vi "Get SMO HELP.vi"(8 "error in (no error)":errorcluster, 10 "Command":string, 11 "Instrument in":refnum<class "Instrument.lvclass">) -> (0 "error out":errorcluster, 2 "help cluster":T1, 3 "Instrument out":refnum<class "Instrument.lvclass">)   [LabVIEW 2019, in "Instrument.lvlib" / "Instrument.lvclass"]
uses:
  Instrument.lvclass
  subsystems/Help/typedefs/Help--cluster.ctl
  Typedefs/Instrument.Commands--Enum.ctl
  Typedefs/Instrument.IDN--cluster.ctl
  Typedefs/Instrument.GET--cluster.ctl
  Typedefs/Instrument.SET--cluster.ctl
  Typedefs/Instrument.HELP--Cluster.ctl
  subsystems/Help/Help.lvclass
  <vilib>/PRIrvin/JSON-Schema/JSON-Schema.lvlib
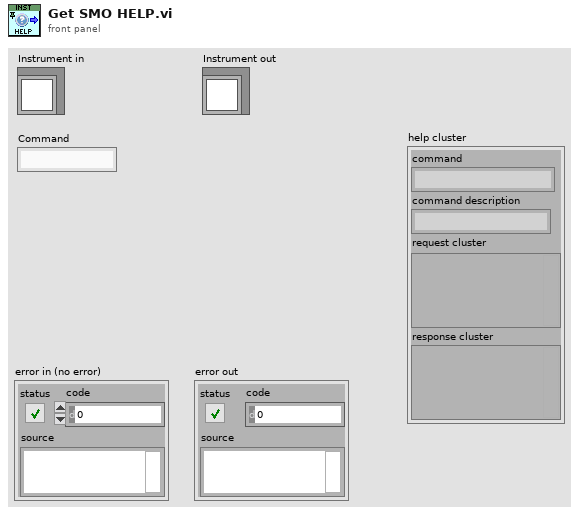
[diagram p1: front panel]
types:
  T1 = typedef "Instrument.lvlib/Help.lvclass/Help--cluster.ctl" = cluster{"command":string, "command description":string, "request cluster":variant, "response cluster":variant}
  T2 = typedef "Instrument.lvlib/Instrument.lvclass/Instrument.GET--cluster.ctl" = cluster{"parameter":string, "Data":variant}
  T3 = typedef "Instrument.lvlib/Instrument.lvclass/Instrument.SET--cluster.ctl" = cluster{"parameter":string, "Data":variant}
  T4 = typedef "Instrument.lvlib/Instrument.lvclass/Instrument.HELP--Cluster.ctl" = cluster{"command":string}
  T5 = typedef "Instrument.lvlib/Instrument.lvclass/Instrument.Commands--Enum.ctl" = enum16{"ACK", "HELP", "IDN", "getAll", "getAllData"}
  T6 = typedef "Instrument.lvlib/Instrument.lvclass/Instrument.IDN--cluster.ctl" = cluster{"vendor":string, "model":string, "serial":string, "firmware":string}
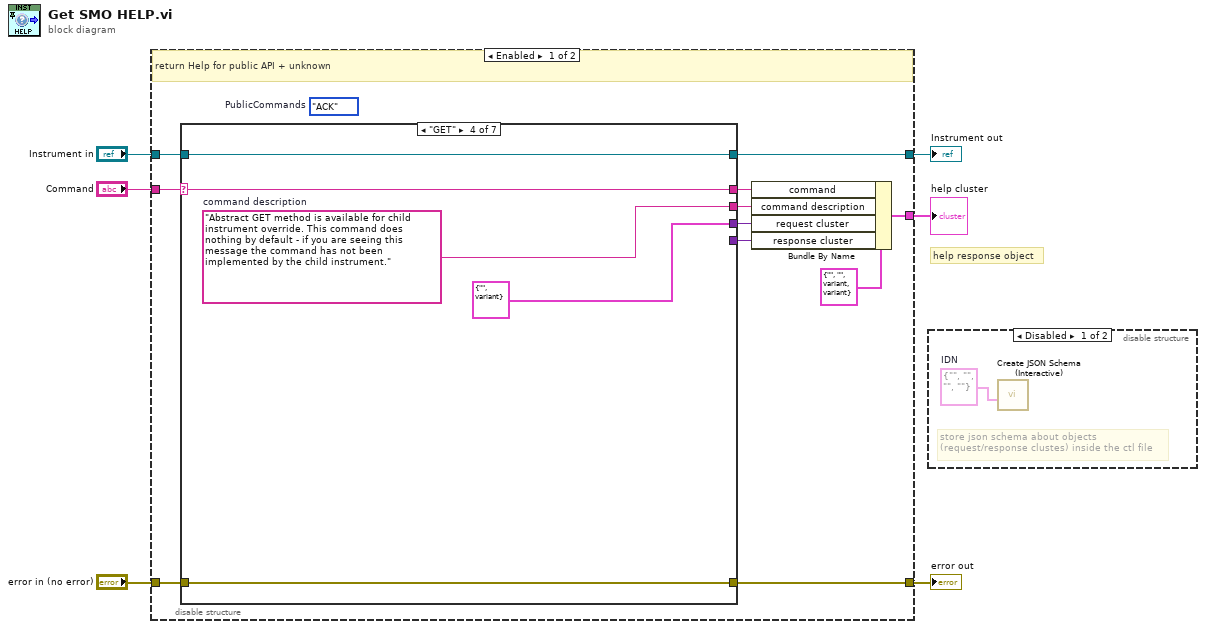
[diagram p0: block diagram]
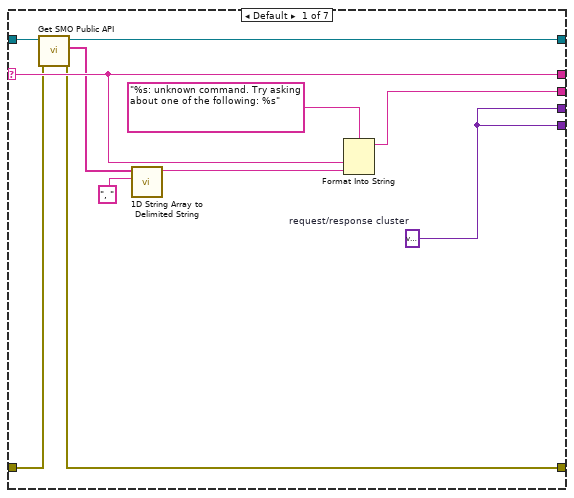
[diagram p3: hidden frame]
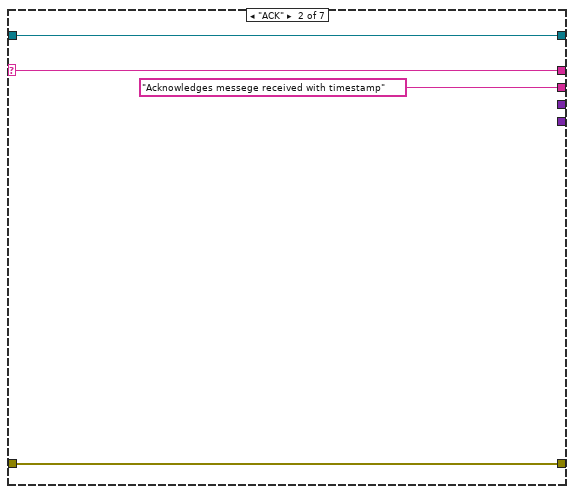
[diagram p4: hidden frame]
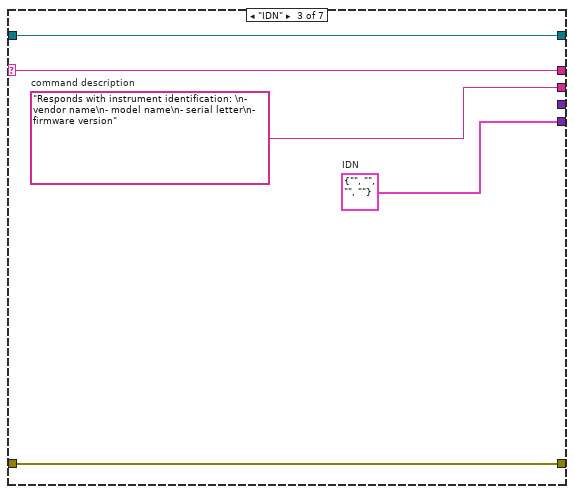
[diagram p5: hidden frame]
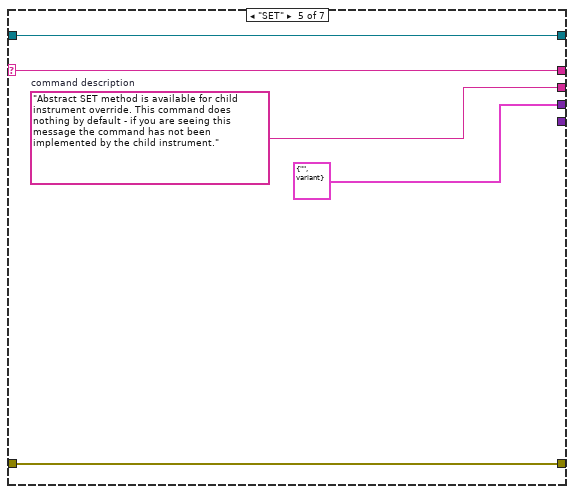
[diagram p6: hidden frame]
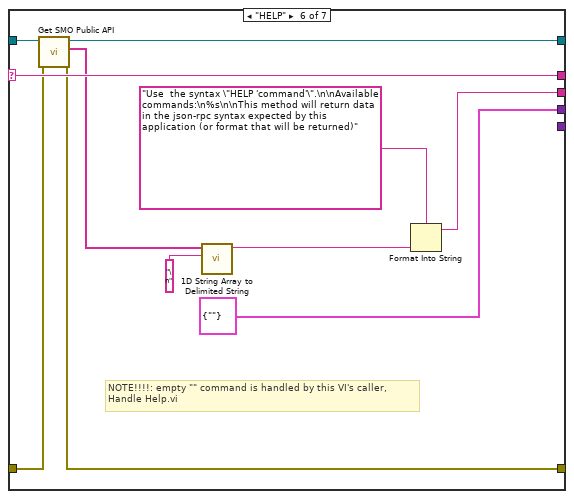
[diagram p7: hidden frame]
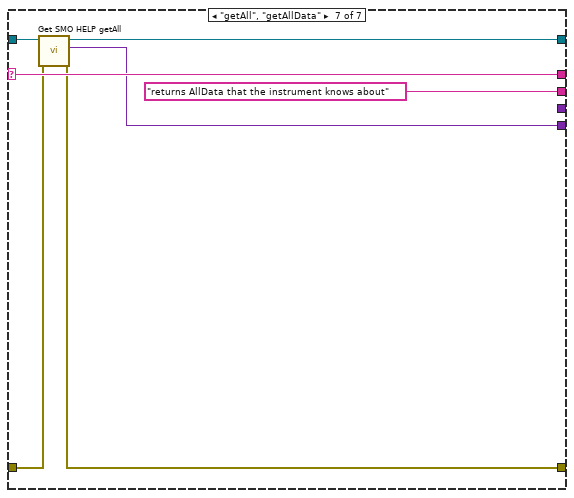
[diagram p8: hidden frame]
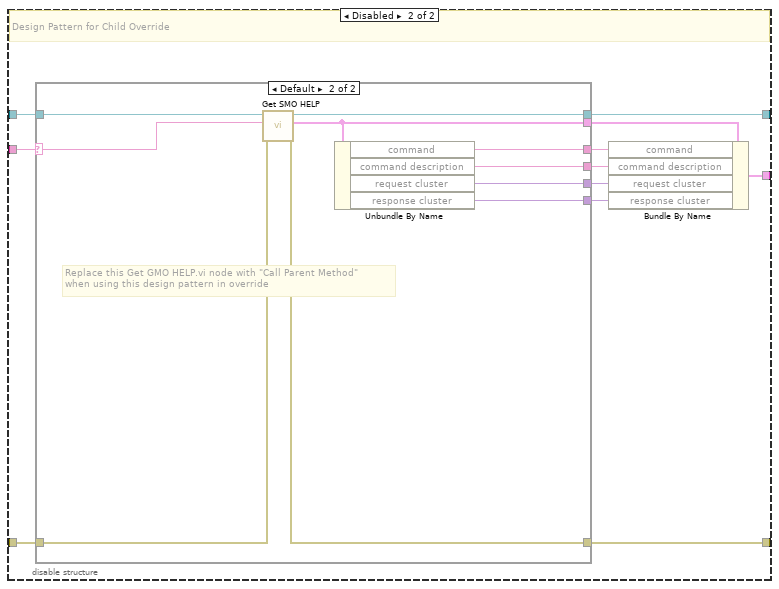
[diagram p9: hidden frame]
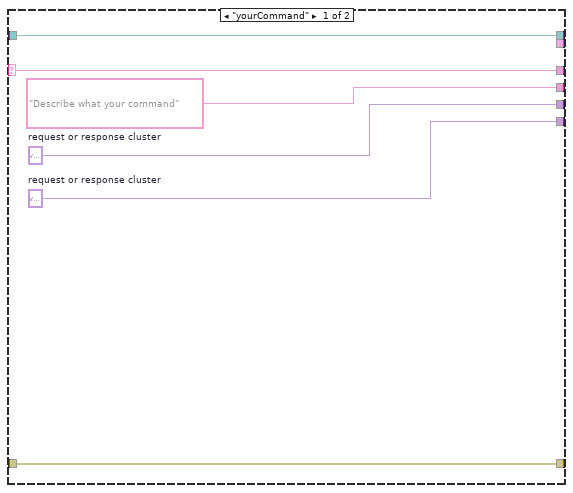
[diagram p10: hidden frame]
diagram:
  # "help response object"
  n1 = disable-structure shown="Enabled" {
    disable-tunnel: [w17 w67] -> w6
    disable-tunnel: "Instrument in" -> [w16 w68]
    disable-tunnel: "error in (no error)" -> [w15 w74]
    disable-tunnel: [w11 w76] -> w3
    disable-tunnel: [w8 w75] -> w2
    disable-tunnel: "Command" -> [w7 w73]
    frame Enabled {
      (unwired) Instrument.Commands--Enum."ACK"  # PublicCommands
      # "return Help for public API + unknown"
      n2 = case shown="\"GET\"" w7 {
        selector: w7 -> [w24 w30 w36 w41 w46 w55 w64]
        tunnel: w15 -> [w21 w32 w34 w39 w44 w52 w63]
        tunnel: [w22 w32 w34 w39 w44 w53 w62] -> w11
        tunnel: [w26 "Acknowledges messege received with timestamp" w37 w42 w47 w49 "returns AllData that the instrument knows about"] -> w13
        tunnel: [w19 _ _ T2 {"parameter"="", "Data"=variant} ("GET") T3 {"parameter"="", "Data"=variant} ("SET") T4 {"command"=""} ("Cluster") _] -> w12
        tunnel: [w19 _ w33 _ _ _ w60] -> w10
        tunnel: [w24 w30 w36 w41 w46 w55 w64] -> w14
        tunnel: w16 -> [w23 w29 w35 w40 w45 w54 w61]
        tunnel: [w20 w29 w35 w40 w45 w51 w59] -> w17
        frame Default {
          w19 = variant  # request/response cluster
          n3 = call-dynamic "Get SMO Public API.vi"("error in (no error)"=w21, "Instrument in"=w23) -> ("error out"=w22:errorcluster, "commands"=w18:string[], "Instrument out"=w20:refnum<class "Instrument.lvclass">)  [unwired: 7 in]
          n4 = call <vilib>:"1D String Array to Delimited String.vi"("delimiter"=", ", "string array"=w18) -> ("delimited string"=w27:string)  [unwired: 9 in]
          n5 = Format Into String(format string="%s: unknown command. Try asking about one of the following: %s", w24, w27) -> (resulting string=w26:string)  [unwired: 2 in, 1 out]
        }
        frame "ACK" {
        }
        frame "IDN" {
          w33 = T6 {"vendor"="", "model"="", "serial"="", "firmware"=""}  # IDN
          w37 = "Responds with instrument identification: \n- vendor name\n- model name\n- serial letter\n- firmware version"  # command description
        }
        frame "GET" {
          w42 = "Abstract GET method is available for child instrument override. This command does nothing by default - if you are seeing this message the command has not been implemented by the child instrument."  # command description
        }
        frame "SET" {
          w47 = "Abstract SET method is available for child instrument override. This command does nothing by default - if you are seeing this message the command has not been implemented by the child instrument."  # command description
        }
        frame "HELP" {
          # "NOTE!!!!: empty \"\" command is handled by this VI's caller,\nHandle Help.vi"
          n6 = call-dynamic "Get SMO Public API.vi"("error in (no error)"=w52, "Instrument in"=w54) -> ("error out"=w53:errorcluster, "commands"=w50:string[], "Instrument out"=w51:refnum<class "Instrument.lvclass">)  [unwired: 7 in]
          n7 = call <vilib>:"1D String Array to Delimited String.vi"("delimiter"="\n", "string array"=w50) -> ("delimited string"=w58:string)  [unwired: 9 in]
          n8 = Format Into String(format string="Use  the syntax \"HELP 'command'\".\n\nAvailable commands:\n%s\n\nThis method will return data in the json-rpc syntax expected by this application (or format that will be returned)", w58) -> (resulting string=w49:string)  [unwired: 2 in, 1 out]
        }
        frame "getAll", "getAllData" {
          n9 = call-dynamic "Get SMO HELP getAll.vi"("error in (no error)"=w63, "Instrument in"=w61) -> ("error out"=w62:errorcluster, "getAll response cluster"=w60:variant, "Instrument out"=w59:refnum<class "Instrument.lvclass">)  [unwired: 7 in]
        }
      }
      n10 = Bundle By Name(cluster=T1 {"command"="", "command description"="", "request cluster"=variant, "response cluster"=variant} ("Help"), "command"=w14, "command description"=w13, "request cluster"=w12, "response cluster"=w10) -> (w8:T1)
    }
    frame Disabled {
      # "Design Pattern for Child Override"
      n11 = case shown="Default" w73 {
        selector: w73 -> [w82 w91]
        tunnel: [w82 w86] -> w72
        tunnel: w74 -> [w81 w84]
        tunnel: [w81 w83] -> w76
        tunnel: ["Describe what your command" w87] -> w71
        tunnel: [w79 w88] -> w70
        tunnel: [w78 w89] -> w69
        tunnel: w68 -> [w77 w92]
        tunnel: [w77 w90] -> w67
        tunnel: [_ w85] -> w66
        frame "yourCommand" {
          w79 = variant  # request or response cluster
          w78 = variant  # request or response cluster
        }
        frame Default {
          # "Replace this Get GMO HELP.vi node with \"Call Parent Method\"\nwhen using this design pattern in override"
          n12 = call-dynamic "Get SMO HELP.vi"("error in (no error)"=w84, "Command"=w91, "Instrument in"=w92) -> ("error out"=w83:errorcluster, "help cluster"=w85:T1, "Instrument out"=w90:refnum<class "Instrument.lvclass">)  [unwired: 6 in]
          n13 = Unbundle By Name(w85) -> ("command"=w86:string, "command description"=w87:string, "request cluster"=w88:variant, "response cluster"=w89:variant)
        }
      }
      n14 = Bundle By Name(cluster=w66, "command"=w72, "command description"=w71, "request cluster"=w70, "response cluster"=w69) -> (w75:T1)
    }
  }
  "Instrument out" <- w6
  "help cluster" <- w2
  "error out" <- w3
  n15 = disable-structure shown="Disabled" {
    frame Disabled {
      w93 = T6 {"vendor"="", "model"="", "serial"="", "firmware"=""}  # IDN
      # "store json schema about objects\n(request/response clustes) inside the ctl file"
      n16 = call <vilib>:"Create JSON Schema (Interactive).vi"("LV Object"=w93) -> ()  [unwired: 9 in, 2 out]
    }
    frame Enabled {
    }
  }
